vi "LED_current_stability.vi"() -> ()   [LabVIEW 2012]
uses:
  <instrlib>/Keithley 2600 Series/Public/Channel.ctl
  <vilib>/Utility/file.llb/Read From Spreadsheet File (DBL).vi
  <vilib>/Utility/file.llb/Write To Spreadsheet File (string).vi
  <vilib>/Utility/file.llb/Write To Spreadsheet File (DBL).vi
  <instrlib>/Keithley 2600 Series/Keithley 2600 Series.lvlib
  <vilib>/Analysis/NI_AALPro.lvlib
  <vilib>/gmath/NI_Gmath.lvlib
panel:
  out "CurDen array":string[](array[string])
  out "power array":string[](array[string])
  out "Power(W)":dbl
  out "DeltaWL":dbl[](array[numeric])
  out "data path":path
  out "DarkSpectrum path":path
  out "Info path":path
  out "AllSpectrum path":path
  out "EQE array":string[](array[string])
  out "LPE array":string[](array[string])
  out "CE array":string[](array[string])
  out "L/L0 array":string[](array[string])
  out "Lum array":string[](array[string])
  out "voltage array":string[](array[string])
  out "current array":string[](array[string])
  out "time array":string[](array[string])
  out "Info3":string
  out "Info2":string
  out "Info1":string
  out "time string":string
  out "date string":string
  out "Status":string
  in  "Tab Control":T1(tab)
  in  "VISA resource name":refnum<visa-resource-name>
  in  "Source Current (A)":dbl=1.1e-05 format="%#_5e"
  in  "Voltage Limit (V)":dbl=10.0
  in  "Integration Time (ms)":dbl=10.0
  in  "Interval (s)":u32=5
  in  "Initial wait (ms)":u32=2000
  in  "Calibration File":path
  in  "Dev_Area (m2)":dbl=3e-06
  in  "WL_high":dbl=785.0
  in  "WL_low":dbl=365.0
  in  "Ratio for auto stop":dbl
  in  "File Path":path
  in  "Auto stop":bool
  in  "Boxcar Width":i32
  in  "Sample description:":string="Please write here..."
  out "Measured Voltage (V)":string
  out "Measured Current (A)":string
  out "WL_2":dbl format="%#_5g"
  out "WL_1":dbl format="%#_5g"
  out "EQE (%)":dbl format="%_3e"
  out "Lum. Pow. Eff. (lm/W)":dbl format="%_3e"
  out "Lum.(cd/m2)":dbl format="%_3e"
  out "Cur. Eff. (cd/A)":dbl format="%_3e"
  out "Lum0":dbl format="%_3e"
  out "Lum/Lum0":dbl format="%_3e"
  out "Time (s)":dbl
  out "Spectra":T2(graph)
  out "Graph":cluster{dbl[], dbl[]}(graph)
  out "Measured_Current(A)":dbl format="%_3e"
  out "Measured_voltage(V)":dbl format="%_3e"
  in  "Ring":i32(ring)=1 items=["L/L0", "Lum", "C.E.", "L.P.E.", "EQE", "Power"]
  out "Maximum Intensity":i32 format="%.2e"
  out "BoxcarWidth":i32
  out "Detector Saturated":bool
  out "All Info":string
  out "VISA resource name out":refnum<visa-resource-name>
  out "error out":errorcluster
  out "x2":i32
  out "x1":i32
  out "Photon_count":dbl
  out "Energy_WL":dbl[](array[numeric])
  out "Candela":dbl
  out "Abs_Irr (W/nm)":dbl[](array[numeric])
  out "Dark_spectrum":dbl[](array[numeric])
  out "Keithley":bool
  out "Spectrometer":bool
  out "Current density (mA/cm2)":dbl
  out "Iso. Coef. itpl":dbl[](array[numeric]) format="%_6g"
  out "WL itpl":dbl[](array[numeric]) format="%_6g"
  out "EyeRespCoef.":dbl[](array[numeric])
  out "WL_EyeResp":dbl[](array[numeric])
  out "WL_cal":dbl[](array[numeric])
  out "cal_CountsToAbsIrr":dbl[](array[numeric])
  in  "Start":bool
  in  "stop":bool
  out "Measured_Spectrum":dbl[](array[numeric])
  out "Wrapper Out":u64
  out "WL_spectrometer":dbl[](array[numeric])
  out "Number of Spectrometers":i32
  out "Node Out":string
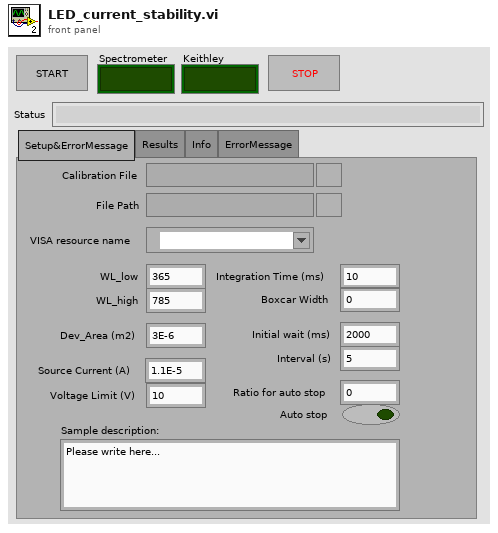
[diagram p1: front panel]
types:
  T1 = enum32{"Setup&ErrorMessage", "Results", "Info", "ErrorMessage"}
  T2 = cluster{"WL_spectrometer":dbl[], "Dark_spectrum":dbl[]}
  T3 = enum32{"Current", "Voltage", "IV", "Resistance", "Power"}
  T4 = typedef "Keithley 2600 Series.lvlib/Channel.ctl" = enum32{"Channel A", "Channel B"}
  T5 = cluster{"WL_spectrometer":dbl[], "Measured_Spectrum":dbl[]}
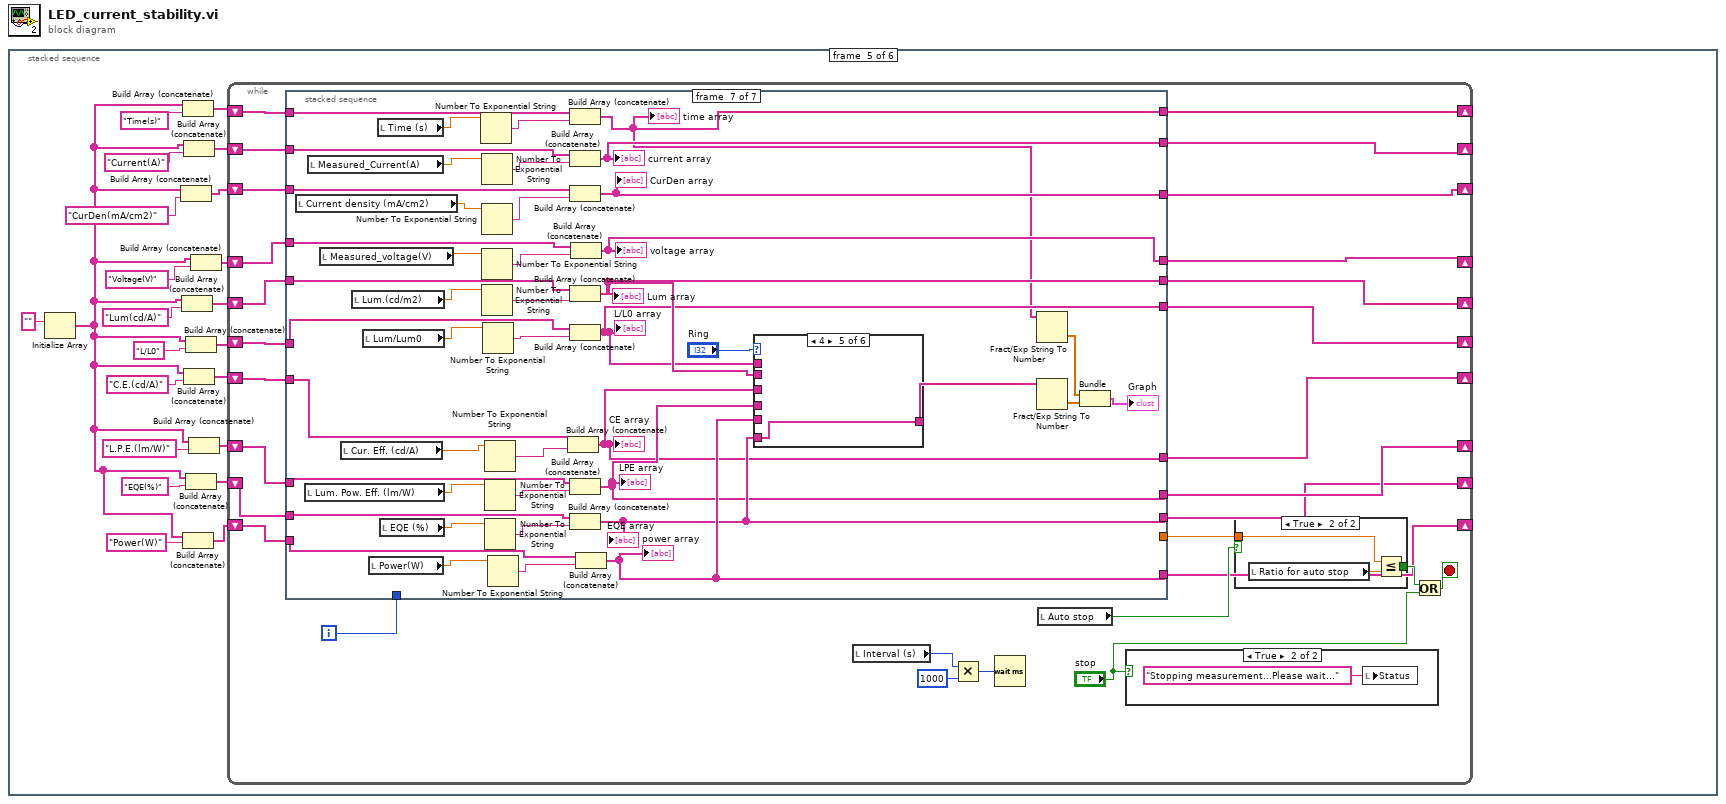
[diagram p0: block diagram]
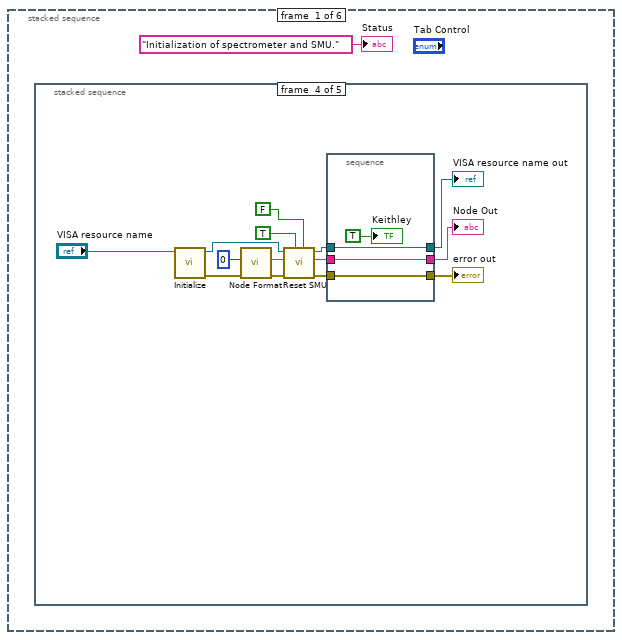
[diagram p2: hidden frame]
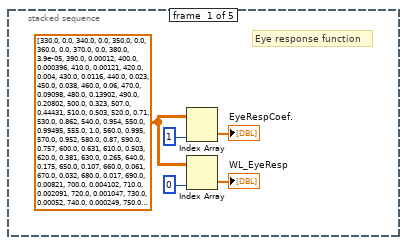
[diagram p3: hidden frame]
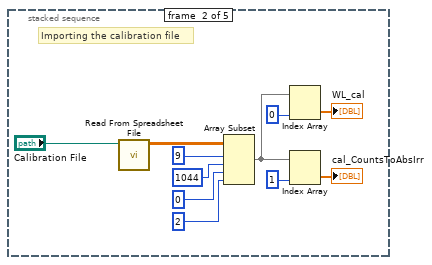
[diagram p4: hidden frame]
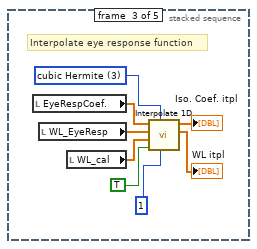
[diagram p5: hidden frame]
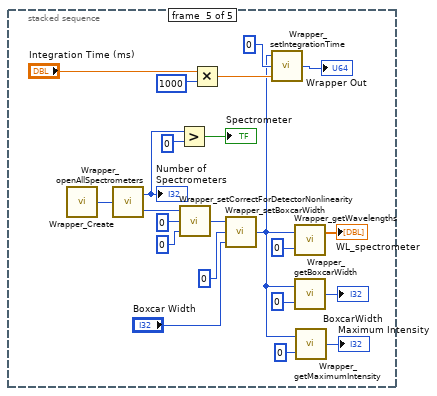
[diagram p6: hidden frame]
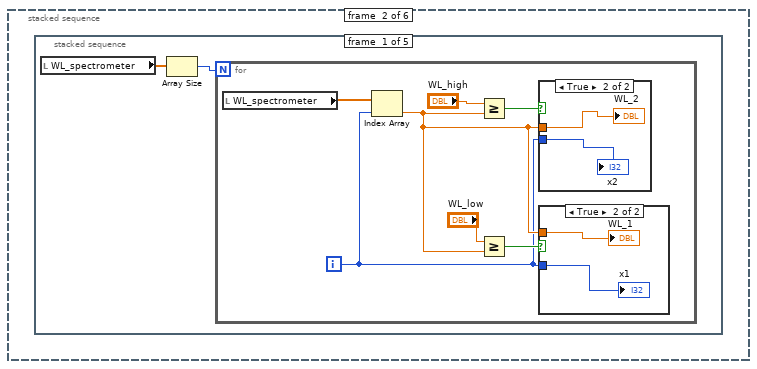
[diagram p7: hidden frame]
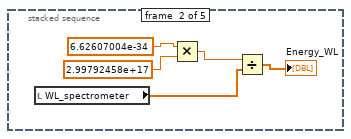
[diagram p10: hidden frame]
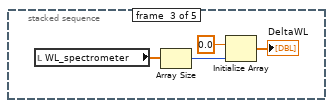
[diagram p11: hidden frame]
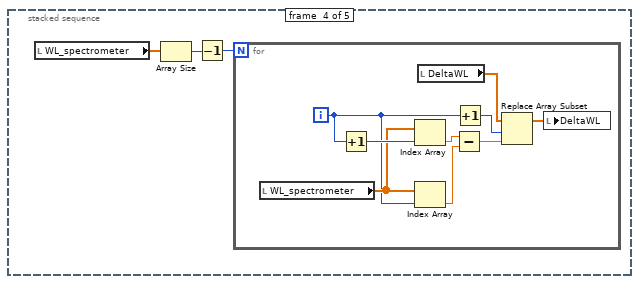
[diagram p12: hidden frame]
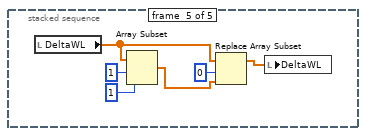
[diagram p13: hidden frame]
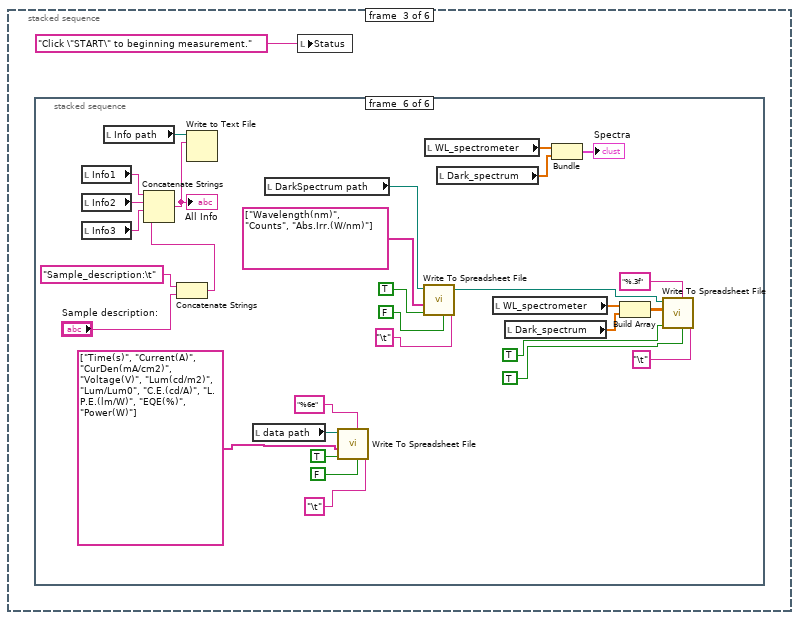
[diagram p14: hidden frame]
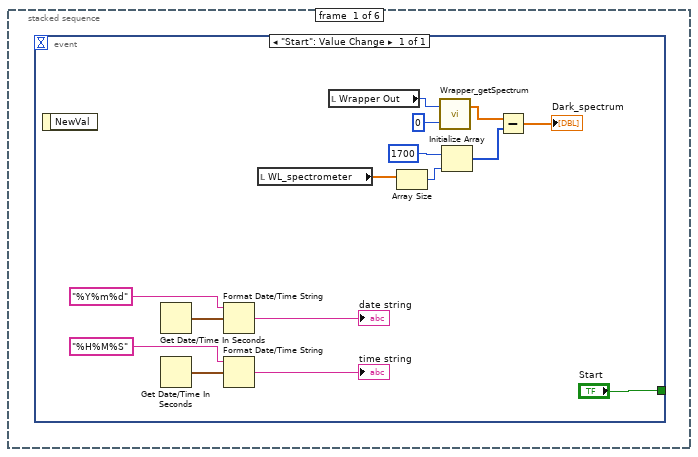
[diagram p15: hidden frame]
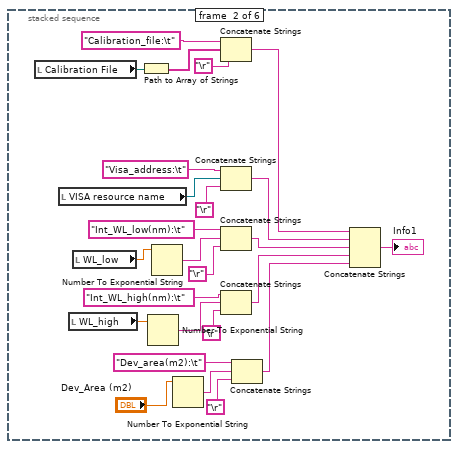
[diagram p16: hidden frame]
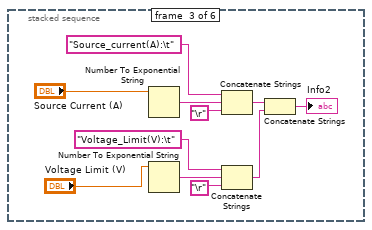
[diagram p17: hidden frame]
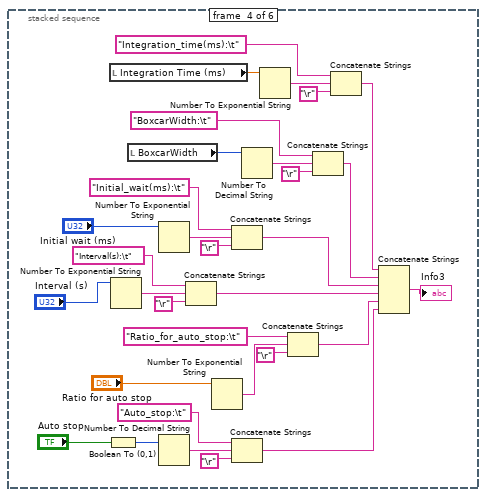
[diagram p18: hidden frame]
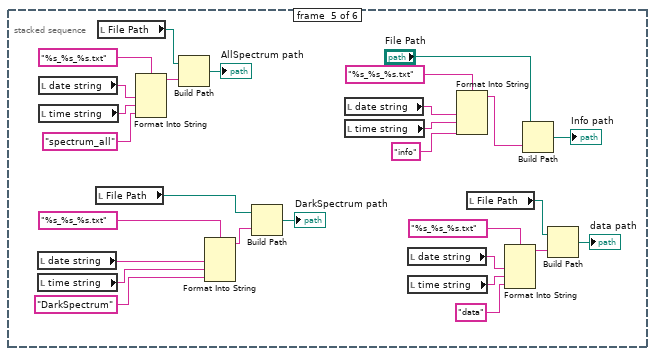
[diagram p19: hidden frame]
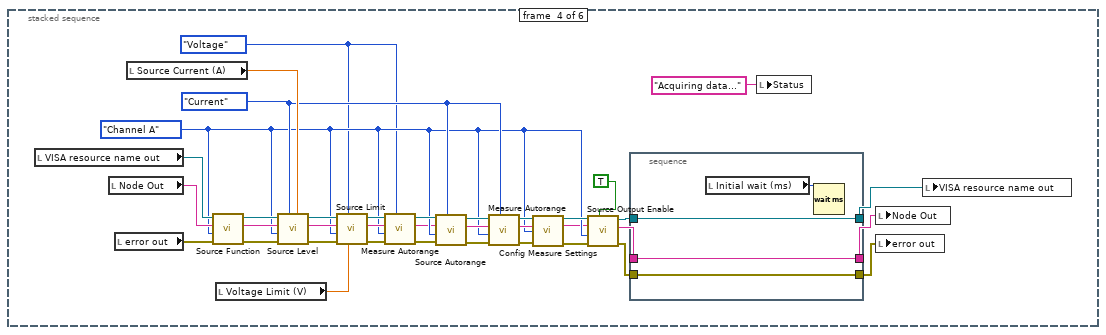
[diagram p20: hidden frame]
diagram:
  n1 = stacked-sequence {
    frame #0 {
      n2 = stacked-sequence {
        frame #0 {
          w5 = dbl[][] [[330.0, 0.0], [340.0, 0.0], [350.0, 0.0], [360.0, 0.0], [370.0, 0.0], [380.0, 3.9e-05], [390.0, 0.00012], [400.0, 0.000396], [410.0, 0.00121], [420.0, 0.004], [430.0, 0.0116], [440.0, 0.023], [450.0, 0.038], [460.0, 0.06], [470.0, 0.09098], [480.0, 0.13902], [490.0, 0.20802], [500.0, 0.323], [507.0, 0.44431], [510.0, 0.503], [520.0, 0.71], [530.0, 0.862], [540.0, 0.954], [550.0, 0.99495], [555.0, 1.0], [560.0, 0.995], [570.0, 0.952], [580.0, 0.87], [590.0, 0.757], [600.0, 0.631], [610.0, 0.503], [620.0, 0.381], [630.0, 0.265], [640.0, 0.175], [650.0, 0.107], [660.0, 0.061], [670.0, 0.032], [680.0, 0.017], [690.0, 0.00821], [700.0, 0.004102], [710.0, 0.002091], [720.0, 0.001047], [730.0, 0.00052], [740.0, 0.000249], [750.0, 0.00012], [760.0, 6e-05], [770.0, 3e-05], [780.0, 0.0], [790.0, 0.0], [800.0, 0.0], [810.0, 0.0], [820.0, 0.0], [830.0, 0.0], [840.0, 0.0], [850.0, 0.0], [860.0, 0.0], [870.0, 0.0], [880.0, 0.0], [890.0, 0.0], [900.0, 0.0], [910.0, 0.0], [920.0, 0.0], [930.0, 0.0], [940.0, 0.0], [950.0, 0.0], [960.0, 0.0], [970.0, 0.0], [980.0, 0.0], [990.0, 0.0], [1000.0, 0.0], [1010.0, 0.0], [1020.0, 0.0], [1030.0, 0.0], [1040.0, 0.0], [1050.0, 0.0], [1060.0, 0.0], [1070.0, 0.0], [1080.0, 0.0], [1090.0, 0.0], [1100.0, 0.0], [1110.0, 0.0], [1120.0, 0.0], [1130.0, 0.0], [1140.0, 0.0]] ("all rows")
          # "Eye response function"
          n3 = Index Array(array=w5, index (col)=1 ("disabled index (col)")) -> (element=→"EyeRespCoef.":dbl[])  [unwired: 1 in]
          n4 = Index Array(array=w5, index (col)=0 ("disabled index (col)")) -> (element=→"WL_EyeResp":dbl[])  [unwired: 1 in]
        }
        frame #1 {
          # "Importing the calibration file"
          n5 = call-poly <vilib>:"Read From Spreadsheet File.vi"("file path (dialog if empty)"="Calibration File") -> ("all rows"=w10:dbl[][])  [unwired: 6 in, 4 out]
          n6 = Array Subset(array=w10, index (row)=9 ("index"), length (row)=1044 ("length"), index (col)=0 ("index"), length (col)=2 ("length")) -> (w13:dbl[][])
          n7 = Index Array(array=w13, index (col)=0 ("index")) -> (element=→"WL_cal":dbl[])  [unwired: 1 in]
          n8 = Index Array(array=w13, index (col)=1 ("length")) -> (element=→"cal_CountsToAbsIrr":dbl[])  [unwired: 1 in]
        }
        frame #2 {
          w21 = 3 items=["nearest", "linear", "spline", "cubic Hermite", "Lagrange"] ("method")
          # "Interpolate eye response function"
          n9 = local read "EyeRespCoef."() -> (w24:dbl[])
          n10 = local read "WL_EyeResp"() -> (w25:dbl[])
          n11 = local read "WL_cal"() -> (w23:dbl[])
          n12 = call <vilib>:"Interpolate 1D.vi"("ntimes"=1, "method"=w21, "X is monotonic"=TRUE, "xi"=w23, "X"=w25, "Y"=w24) -> ("xi used"=→"WL itpl":dbl[], "yi"=→"Iso. Coef. itpl":dbl[])  [unwired: 3 in, 1 out]
        }
        frame #3 {
          n13 = call <instrlib>:"Initialize.vi"("VISA resource name"="VISA resource name") -> ("error out"=w37:errorcluster, "VISA resource name out"=w39:refnum<visa-resource-name>)  [unwired: 5 in, 4 out]
          n14 = call <instrlib>:"Node Format.vi"("error in"=w37, "Node (0-64)"=i8 0) -> ("error out"=w36:errorcluster, "Formatted Node"=w38:string)  [unwired: 8 out]
          n15 = call <instrlib>:"Reset SMU.vi"("SMU B (No)"=FALSE, "SMU A (No)"=TRUE, "error in (no error)"=w36, "Node In"=w38, "VISA resource name"=w39) -> ("error out"=w31:errorcluster, "Node Out"=w29:string, "VISA resource name out"=w27:refnum<visa-resource-name>)  [unwired: 4 out]
          n16 = stacked-sequence {
            tunnel: [w42] -> w30
            tunnel: w31 -> [w42]
            tunnel: w29 -> [w41]
            tunnel: [w41] -> w28
            tunnel: w27 -> [w40]
            tunnel: [w40] -> w26
            frame #0 {
              "Keithley" <- TRUE ("Keithley")
            }
          }
          "Node Out" <- w28
          "error out" <- w30
          "VISA resource name out" <- w26
        }
        frame #4 {
          n17 = call "Wrapper_Create.vi"() -> ("Wrapper"=w65:u64)
          n18 = call "Wrapper_openAllSpectrometers.vi"("Wrapper In"=w65) -> ("Number of Spectrometers"=w58:i32, "Wrapper Out"=w49:u64)
          "Number of Spectrometers" <- w58
          n19 = Greater?(x=w58, y=0) -> (0:→"Spectrometer":bool)
          n20 = call "Wrapper_setCorrectForDetectorNonlinearity.vi"("On/Off"=0, "Index"=0, "Wrapper In"=w49) -> ("Wrapper Out"=w54:u64)
          n21 = Multiply(x="Integration Time (ms)", y=1000) -> (x*y=w61:dbl)
          n22 = call "Wrapper_setBoxcarWidth.vi"("Boxcar Width"="Boxcar Width", "Index"=0, "Wrapper In"=w54) -> ("Wrapper Out"=w48:u64)
          n23 = call "Wrapper_setIntegrationTime.vi"("Integration Time"=w61, "Index"=0, "Wrapper In"=w48) -> ("Wrapper Out"=→"Wrapper Out":u64)
          n24 = call "Wrapper_getWavelengths.vi"("Index"=0, "Wrapper"=w48) -> ("WL Values"=→"WL_spectrometer":dbl[])  [unwired: 1 out]
          n25 = call "Wrapper_getBoxcarWidth.vi"("Index"=0, "Wrapper"=w48) -> ("BoxcarWidth"=→"BoxcarWidth":i32)
          n26 = call "Wrapper_getMaximumIntensity.vi"("Index"=0, "Wrapper"=w48) -> ("Maximum Intensity"=→"Maximum Intensity":i32)
        }
      }
      "Status" <- "Initialization of spectrometer and SMU." ("Measured Current (A) 2")
    }
    frame #1 {
      n27 = stacked-sequence {
        frame #0 {
          n28 = local read "WL_spectrometer"() -> (w66:dbl[])
          n29 = Array Size(array=w66) -> (size(s)=w67:i32)
          n30 = for {
            N: w67 -> [_]
            i -> [w68]
            n31 = local read "WL_spectrometer"() -> (w70:dbl[])
            n32 = Index Array(array=w70, index=w68) -> (element=w69:dbl)
            n33 = Greater Or Equal?(x="WL_high", y=w69) -> (x >= y?=w72:bool)
            n34 = Greater Or Equal?(x="WL_low", y=w69) -> (x >= y?=w71:bool)
            n35 = case shown="True" w72 {
              tunnel: w69 -> [_ w77]
              tunnel: w68 -> [_ w78]
              frame False {
              }
              frame True {
                "WL_2" <- w77
                "x2" <- w78
              }
            }
            n36 = case shown="True" w71 {
              tunnel: w69 -> [_ w75]
              tunnel: w68 -> [_ w76]
              frame False {
              }
              frame True {
                "WL_1" <- w75
                "x1" <- w76
              }
            }
          }
        }
        frame #1 {
          n37 = local read "WL_spectrometer"() -> (w82:dbl[])
          n38 = Multiply(x=6.62607004e-34, y=2.99792458e+17) -> (x*y=w81:dbl)
          n39 = Divide(x=w81, y=w82) -> (x/y=→"Energy_WL":dbl[])
        }
        frame #2 {
          n40 = local read "WL_spectrometer"() -> (w87:dbl[])
          n41 = Array Size(array=w87) -> (size(s)=w85:i32)
          n42 = Initialize Array(0.0, w85) -> (→"DeltaWL":dbl[])
        }
        frame #3 {
          n43 = local read "WL_spectrometer"() -> (w90:dbl[])
          n44 = Array Size(array=w90) -> (size(s)=w89:i32)
          n45 = Decrement(x=w89) -> (x-1=w88:i32)
          n46 = for {
            N: w88 -> [_]
            i -> [w95]
            n47 = local read "WL_spectrometer"() -> (w98:dbl[])
            n48 = Increment(x=w95) -> (x+1=w99:i32)
            n49 = Index Array(array=w98, index=w99) -> (element=w97:dbl)
            n50 = Index Array(array=w98, index=w95) -> (element=w96:dbl)
            n51 = local read "DeltaWL"() -> (w92:dbl[])
            n52 = Subtract(x=w97, y=w96) -> (x-y=w93:dbl)
            n53 = Increment(x=w95) -> (x+1=w94:i32)
            n54 = Replace Array Subset(array=w92, new element=w93, index=w94) -> (w91:dbl[])
            n55 = local write "DeltaWL"(w91) -> ()
          }
        }
        frame #4 {
          n56 = local read "DeltaWL"() -> (w100:dbl[])
          n57 = Array Subset(array=w100, index=1, length=1) -> (w101:dbl[])
          n58 = Replace Array Subset(array=w100, new element=w101, index=0) -> (w105:dbl[])
          n59 = local write "DeltaWL"(w105) -> ()
        }
      }
    }
    frame #2 {
      n60 = stacked-sequence {
        frame #0 {
          n61 = event shown="[0] \"Start\": Value Change" {
            selector: _ -> [_]
            dyn-events: _ -> [_]
            timeout: _ -> [_]
            tunnel: ["Start"] -> _
            event "Start": Value Change {
              n62 = event-data() -> ()  [unwired: 1 in, 1 out]
              n63 = Get Date/Time In Seconds() -> (seconds since 1Jan1904=w119:timestamp)
              n64 = Get Date/Time In Seconds() -> (seconds since 1Jan1904=w117:timestamp)
              n65 = Format Date/Time String(time format string (%c)="%Y%m%d" ("Timestamp string format i%cj"), seconds (now)=w119) -> (date/time string=→"date string":string)  [unwired: 1 out]
              n66 = Format Date/Time String(time format string (%c)="%H%M%S" ("Timestamp string format i%cj"), seconds (now)=w117) -> (date/time string=→"time string":string)  [unwired: 1 out]
              n67 = local read "WL_spectrometer"() -> (w112:dbl[])
              n68 = local read "Wrapper Out"() -> (w113:u64)
              n69 = Array Size(array=w112) -> (size(s)=w111:i32)
              n70 = call "Wrapper_getSpectrum.vi"("Index"=0, "Wrapper"=w113) -> ("Spectrum Values"=w109:dbl[])  [unwired: 1 out]
              n71 = Initialize Array(1700, w111) -> (w108:i32[])
              n72 = Subtract(x=w109, y=w108) -> (x-y=→"Dark_spectrum":dbl[])
            }
          }
        }
        frame #1 {
          n73 = local read "Calibration File"() -> (w123:path)
          n74 = local read "VISA resource name"() -> (w129:refnum<visa-resource-name>)
          n75 = local read "WL_high"() -> (w125:dbl)
          n76 = local read "WL_low"() -> (w124:dbl)
          n77 = Path to Array of Strings(0:w123) -> (2:w127:string[])  [unwired: 1 out]
          n78 = Number To Exponential String(number=w125) -> (E-format string=w133:string)  [unwired: 3 in]
          n79 = Number To Exponential String(number=w124) -> (E-format string=w130:string)  [unwired: 3 in]
          n80 = Number To Exponential String(number="Dev_Area (m2)") -> (E-format string=w136:string)  [unwired: 3 in]
          n81 = Concatenate Strings("Calibration_file:\t" ("string"), w127, "\r") -> (w137:string)
          n82 = Concatenate Strings("Visa_address:\t" ("string"), w129, "\r") -> (w138:string)
          n83 = Concatenate Strings("Int_WL_low(nm):\t" ("string"), w130, "\r") -> (w139:string)
          n84 = Concatenate Strings("Int_WL_high(nm):\t" ("string"), w133, "\r") -> (w140:string)
          n85 = Concatenate Strings("Dev_area(m2):\t" ("string"), w136, "\r") -> (w141:string)
          n86 = Concatenate Strings(w137, w138, w139, w140, w141) -> (→"Info1":string)
        }
        frame #2 {
          n87 = Number To Exponential String(number="Source Current (A)") -> (E-format string=w149:string)  [unwired: 3 in]
          n88 = Number To Exponential String(number="Voltage Limit (V)") -> (E-format string=w152:string)  [unwired: 3 in]
          n89 = Concatenate Strings("Source_current(A):\t" ("string"), w149, "\r") -> (w154:string)
          n90 = Concatenate Strings("Voltage_Limit(V):\t" ("string"), w152, "\r") -> (w155:string)
          n91 = Concatenate Strings(w154, w155) -> (→"Info2":string)
        }
        frame #3 {
          n92 = Boolean To (0,1)(Boolean="Auto stop") -> (0, 1=w166:i16)
          n93 = local read "Integration Time (ms)"() -> (w177:dbl)
          n94 = Number To Exponential String(number="Interval (s)") -> (E-format string=w183:string)  [unwired: 3 in]
          n95 = local read "BoxcarWidth"() -> (w159:i32)
          n96 = Number To Exponential String(number="Initial wait (ms)") -> (E-format string=w179:string)  [unwired: 3 in]
          n97 = Number To Decimal String(number=w166) -> (decimal integer string=w165:string)  [unwired: 1 in]
          n98 = Concatenate Strings("Interval(s):\t" ("string"), w183, "\r") -> (w188:string)
          n99 = Number To Exponential String(number="Ratio for auto stop") -> (E-format string=w184:string)  [unwired: 3 in]
          n100 = Concatenate Strings("Initial_wait(ms):\t" ("string"), w179, "\r") -> (w187:string)
          n101 = Concatenate Strings("Auto_stop:\t" ("string"), w165, "\r") -> (w164:string)
          n102 = Number To Decimal String(number=w159) -> (decimal integer string=w163:string)  [unwired: 1 in]
          n103 = Number To Exponential String(number=w177) -> (E-format string=w176:string)  [unwired: 3 in]
          n104 = Concatenate Strings("Ratio_for_auto_stop:\t" ("string"), w184, "\r") -> (w189:string)
          n105 = Concatenate Strings("BoxcarWidth:\t" ("string"), w163, "\r") -> (w161:string)
          n106 = Concatenate Strings("Integration_time(ms):\t" ("string"), w176, "\r") -> (w160:string)
          n107 = Concatenate Strings(w160, w161, w187, w188, w189, w164) -> (→"Info3":string)
        }
        frame #4 {
          n108 = local read "date string"() -> (w203:string)
          n109 = local read "time string"() -> (w204:string)
          n110 = local read "date string"() -> (w214:string)
          n111 = local read "time string"() -> (w215:string)
          n112 = local read "File Path"() -> (w202:path)
          n113 = local read "File Path"() -> (w216:path)
          n114 = Format Into String(format string="%s_%s_%s.txt" ("Format string"), w214, w215, "spectrum_all" ("input 2")) -> (resulting string=w213:string)  [unwired: 2 in, 1 out]
          n115 = Build Path(base path=w216, name or relative path=w213) -> (appended path=→"AllSpectrum path":path)
          n116 = Format Into String(format string="%s_%s_%s.txt" ("Format string"), w203, w204, "DarkSpectrum" ("input 2")) -> (resulting string=w201:string)  [unwired: 2 in, 1 out]
          n117 = Build Path(base path=w202, name or relative path=w201) -> (appended path=→"DarkSpectrum path":path)
          n118 = local read "date string"() -> (w207:string)
          n119 = local read "time string"() -> (w209:string)
          n120 = local read "date string"() -> (w192:string)
          n121 = local read "time string"() -> (w193:string)
          n122 = Format Into String(format string="%s_%s_%s.txt" ("Format string"), w207, w209, "info" ("input 2")) -> (resulting string=w210:string)  [unwired: 2 in, 1 out]
          n123 = local read "File Path"() -> (w195:path)
          n124 = Format Into String(format string="%s_%s_%s.txt" ("Format string"), w192, w193, "data" ("input 2")) -> (resulting string=w191:string)  [unwired: 2 in, 1 out]
          n125 = Build Path(base path="File Path", name or relative path=w210) -> (appended path=→"Info path":path)
          n126 = Build Path(base path=w195, name or relative path=w191) -> (appended path=→"data path":path)
        }
        frame #5 {
          n127 = local read "Info1"() -> (w246:string)
          n128 = local read "Info2"() -> (w245:string)
          n129 = local read "Info3"() -> (w244:string)
          n130 = local read "Info path"() -> (w233:path)
          n131 = Concatenate Strings("Sample_description:\t" ("string"), "Sample description:") -> (w218:string)
          n132 = Concatenate Strings(w246, w245, w244, w218) -> (w247:string)
          "All Info" <- w247
          n133 = Write to Text File(file (use dialog)=w233, text=w247) -> ()  [unwired: 2 in, 3 out]
          n134 = local read "data path"() -> (w226:path)
          n135 = local read "DarkSpectrum path"() -> (w228:path)
          n136 = call-poly <vilib>:"Write To Spreadsheet File.vi"("delimiter (\\t)"="\t" ("delimiter (\\t)"), "transpose? (no:F)"=FALSE, "format (%s)"="%6e" ("format (%.3f)"), "append to file? (new file:F)"=TRUE, "1D data"=string[] ["Time(s)", "Current(A)", "CurDen(mA/cm2)", "Voltage(V)", "Lum(cd/m2)", "Lum/Lum0", "C.E.(cd/A)", "L.P.E.(lm/W)", "EQE(%)", "Power(W)"], "file path (dialog if empty)"=w226) -> ()  [unwired: 1 in, 2 out]
          n137 = call-poly <vilib>:"Write To Spreadsheet File.vi"("delimiter (\\t)"="\t" ("delimiter (\\t)"), "transpose? (no:F)"=FALSE, "append to file? (new file:F)"=TRUE, "1D data"=string[] ["Wavelength(nm)", "Counts", "Abs.Irr.(W/nm)"], "file path (dialog if empty)"=w228) -> ("new file path (Not A Path if cancelled)"=w227:path)  [unwired: 2 in, 1 out]
          n138 = local read "WL_spectrometer"() -> (w234:dbl[])
          n139 = local read "Dark_spectrum"() -> (w235:dbl[])
          n140 = local read "WL_spectrometer"() -> (w238:dbl[])
          n141 = local read "Dark_spectrum"() -> (w237:dbl[])
          n142 = Bundle("WL_spectrometer"=w234, "Dark_spectrum"=w235) -> (→"Spectra":T2)  [unwired: 1 in]
          n143 = Build Array(w238, w237) -> (w239:dbl[][])
          n144 = call-poly <vilib>:"Write To Spreadsheet File.vi"("delimiter (\\t)"="\t" ("delimiter (\\t)"), "transpose? (no:F)"=TRUE, "format (%.3f)"="%.3f", "append to file? (new file:F)"=TRUE, "2D data"=w239, "file path (dialog if empty)"=w227) -> ()  [unwired: 1 in, 2 out]
        }
      }
      n145 = local write "Status"("Click \"START\" to beginning measurement." ("Status")) -> ()
    }
    frame #3 {
      w251 = enum32{"Current", "Voltage"}."Voltage" ("Function (Current)")
      w257 = enum32{"Current", "Voltage"}."Current" ("Function (Current)")
      w252 = Channel."Channel A" ("Channel (Channel A)")
      n146 = local read "VISA resource name out"() -> (w276:refnum<visa-resource-name>)
      n147 = local read "Node Out"() -> (w277:string)
      n148 = local read "error out"() -> (w278:errorcluster)
      n149 = local read "Source Current (A)"() -> (w268:dbl)
      n150 = call <instrlib>:"Source Function.vi"("error in (no error)"=w278, "Channel (Channel A)"=w252, "Node In"=w277, "VISA resource name"=w276) -> ("error out"=w281:errorcluster, "Node Out"=w279:string, "VISA resource name out"=w280:refnum<visa-resource-name>)  [unwired: 1 in, 4 out]
      n151 = local read "Voltage Limit (V)"() -> (w267:dbl)
      n152 = call <instrlib>:"Source Level.vi"("Level (0.000)"=w268, "Function (Current)"=w257, "error in (no error)"=w281, "Channel (Channel A)"=w252, "Node In"=w279, "VISA resource name"=w280) -> ("error out"=w282:errorcluster, "Node Out"=w284:string, "VISA resource name out"=w283:refnum<visa-resource-name>)  [unwired: 3 out]
      n153 = call <instrlib>:"Source Limit.vi"("Limit (0.000)"=w267, "Function (Current)"=w251, "error in (no error)"=w282, "Channel (Channel A)"=w252, "Node In"=w284, "VISA resource name"=w283) -> ("error out"=w260:errorcluster, "Node Out"=w259:string, "VISA resource name out"=w258:refnum<visa-resource-name>)  [unwired: 3 out]
      n154 = call <instrlib>:"Measure Autorange.vi"("Function (Current)"=w251, "error in (no error)"=w260, "Channel (Channel A)"=w252, "Node In"=w259, "VISA resource name"=w258) -> ("error out"=w256:errorcluster, "Node Out"=w250:string, "VISA resource name out"=w255:refnum<visa-resource-name>)  [unwired: 1 in, 3 out]
      n155 = call <instrlib>:"Source Autorange.vi"("Function (Current)"=w257, "error in (no error)"=w256, "Channel (Channel A)"=w252, "Node In"=w250, "VISA resource name"=w255) -> ("error out"=w264:errorcluster, "Node Out"=w261:string, "VISA resource name out"=w265:refnum<visa-resource-name>)  [unwired: 1 in, 3 out]
      n156 = call <instrlib>:"Measure Autorange.vi"("Function (Current)"=w257, "error in (no error)"=w264, "Channel (Channel A)"=w252, "Node In"=w261, "VISA resource name"=w265) -> ("error out"=w263:errorcluster, "Node Out"=w262:string, "VISA resource name out"=w266:refnum<visa-resource-name>)  [unwired: 1 in, 3 out]
      n157 = call <instrlib>:"Config Measure Settings.vi"("VISA resource name"=w266, "Node In"=w262, "Channel (Channel A)"=w252, "error in"=w263) -> ("VISA resource name out"=w253:refnum<visa-resource-name>, "Node Out"=w249:string, "error out"=w254:errorcluster)  [unwired: 6 in, 3 out]
      n158 = call <instrlib>:"Source Output Enable.vi"("Output (Off)"=TRUE, "error in (no error)"=w254, "Channel (Channel A)"=w252, "Node In"=w249, "VISA resource name"=w253) -> ("error out"=w274:errorcluster, "Node Out"=w273:string, "VISA resource name out"=w272:refnum<visa-resource-name>)  [unwired: 4 out]
      n159 = stacked-sequence {
        tunnel: w274 -> [w288]
        tunnel: [w288] -> w269
        tunnel: w273 -> [w287]
        tunnel: [w287] -> w270
        tunnel: w272 -> [w286]
        tunnel: [w286] -> w271
        frame #0 {
          n160 = local read "Initial wait (ms)"() -> (w285:u32)
          n161 = Wait (ms)(milliseconds to wait=w285) -> ()  [unwired: 1 out]
        }
      }
      n162 = local write "Status"("Acquiring data..." ("Status")) -> ()
      n163 = local write "Node Out"(w270) -> ()
      n164 = local write "error out"(w269) -> ()
      n165 = local write "VISA resource name out"(w271) -> ()
    }
    frame #4 {
      n166 = Initialize Array("" ("element")) -> (w291:string[])  [unwired: 1 in]
      n167 = Build Array (concatenate)(w291, "CurDen(mA/cm2)" ("Status")) -> (w289:string[])
      n168 = Build Array (concatenate)(w291, "Lum(cd/A)" ("Status")) -> (w298:string[])
      n169 = Build Array (concatenate)(w291, "Time(s)" ("Status")) -> (w295:string[])
      n170 = Build Array (concatenate)(w291, "Power(W)" ("Status")) -> (w290:string[])
      n171 = Build Array (concatenate)(w291, "Current(A)" ("Status")) -> (w296:string[])
      n172 = Build Array (concatenate)(w291, "C.E.(cd/A)" ("Status")) -> (w300:string[])
      n173 = Build Array (concatenate)(w291, "L/L0" ("Status")) -> (w299:string[])
      n174 = Build Array (concatenate)(w291, "EQE(%)" ("Status")) -> (w302:string[])
      n175 = Build Array (concatenate)(w291, "L.P.E.(lm/W)" ("Status")) -> (w301:string[])
      n176 = Build Array (concatenate)(w291, "Voltage(V)" ("Status")) -> (w297:string[])
      n177 = while {
        shift-right: [w325] -> _
        shift-left: w295 -> [w333]
        shift-right: [w324] -> _
        shift-left: w296 -> [w332]
        shift-right: [w323] -> _
        shift-left: w297 -> [w331]
        shift-right: [w322] -> _
        shift-left: w298 -> [w330]
        shift-right: [w321] -> _
        shift-left: w299 -> [w329]
        shift-right: [w320] -> _
        shift-left: w300 -> [w328]
        shift-right: [w318] -> _
        shift-left: w302 -> [w326]
        shift-right: [w319] -> _
        shift-left: w301 -> [w327]
        shift-right: [w315] -> _
        shift-left: w290 -> [w316]
        shift-right: [w313] -> _
        shift-left: w289 -> [w314]
        i -> [w337]
        stop <- w336 stop-if-true
        n178 = stacked-sequence {
          tunnel: w337 -> [_ _ _ w448 _ _ _]
          tunnel: w333 -> [_ _ _ _ _ _ w530]
          tunnel: w332 -> [_ _ _ _ _ _ w529]
          tunnel: w331 -> [_ _ _ _ _ _ w528]
          tunnel: w330 -> [_ _ _ _ _ _ w527]
          tunnel: w329 -> [_ _ _ _ _ _ w526]
          tunnel: w328 -> [_ _ _ _ _ _ w525]
          tunnel: w327 -> [_ _ _ _ _ _ w524]
          tunnel: w326 -> [_ _ _ _ _ _ w523]
          tunnel: [_ _ _ _ _ _ w486] -> w325
          tunnel: [_ _ _ _ _ _ w500] -> w324
          tunnel: [_ _ _ _ _ _ w498] -> w323
          tunnel: [_ _ _ _ _ _ w488] -> w322
          tunnel: [_ _ _ _ _ _ w487] -> w321
          tunnel: [_ _ _ _ _ _ w489] -> w320
          tunnel: [_ _ _ _ _ _ w490] -> w319
          tunnel: [_ _ _ _ _ _ w491] -> w318
          tunnel: w316 -> [_ _ _ _ _ _ w504]
          tunnel: [_ _ _ _ _ _ w492] -> w315
          tunnel: w314 -> [_ _ _ _ _ _ w501]
          tunnel: [_ _ _ _ _ _ w499] -> w313
          tunnel: [_ _ _ _ w467 _ _] -> w312
          frame #0 {
            w363 = Channel."Channel A" ("Channel (Channel A)")
            n179 = local read "VISA resource name out"() -> (w360:refnum<visa-resource-name>)
            n180 = local read "Node Out"() -> (w361:string)
            n181 = local read "error out"() -> (w362:errorcluster)
            n182 = local read "Wrapper Out"() -> (w351:u64)
            n183 = local read "WL_spectrometer"() -> (w348:dbl[])
            n184 = call "Wrapper_getSpectrum.vi"("Index"=0, "Wrapper"=w351) -> ("Spectrum Values"=w346:dbl[])  [unwired: 1 out]
            n185 = Array Size(array=w348) -> (size(s)=w349:i32)
            n186 = call <instrlib>:"Measure.vi"("Function (Current)"=T3."Voltage", "error in (no error)"=w362, "Channel (Channel A)"=w363, "Node In"=w361, "VISA resource name"=w360) -> ("error out"=w371:errorcluster, "Output"=w353:string, "Node Out"=w370:string, "VISA resource name out"=w369:refnum<visa-resource-name>)  [unwired: 2 in, 1 out]
            "Measured Voltage (V)" <- w353
            n187 = Initialize Array(1700, w349) -> (w347:i32[])
            n188 = Fract/Exp String To Number(string=w353) -> (number=→"Measured_voltage(V)":dbl)  [unwired: 3 in, 1 out]
            n189 = Subtract(x=w346, y=w347) -> (x-y=→"Measured_Spectrum":dbl[])
            n190 = call <instrlib>:"Measure.vi"("Function (Current)"=T3."Current", "error in (no error)"=w371, "Channel (Channel A)"=w363, "Node In"=w370, "VISA resource name"=w369) -> ("error out"=w365:errorcluster, "Output"=w356:string, "Node Out"=w367:string, "VISA resource name out"=w366:refnum<visa-resource-name>)  [unwired: 2 in, 1 out]
            "Measured Current (A)" <- w356
            n191 = local write "VISA resource name out"(w366) -> ()
            n192 = local write "Node Out"(w367) -> ()
            n193 = local write "error out"(w365) -> ()
            n194 = local read "Dev_Area (m2)"() -> (w352:dbl)
            n195 = Fract/Exp String To Number(string=w356) -> (number=w357:dbl)  [unwired: 3 in, 1 out]
            "Measured_Current(A)" <- w357
            n196 = Divide(x=w357, y=w352) -> (x/y=w358:dbl)
            n197 = Multiply(x=w358, y=0.1) -> (x*y=→"Current density (mA/cm2)":dbl)
          }
          frame #1 {
            n198 = local read "Integration Time (ms)"() -> (w412:dbl)
            n199 = local read "Measured_Spectrum"() -> (w406:dbl[])
            n200 = local read "Measured_Spectrum"() -> (w415:dbl[])
            n201 = local read "WL_spectrometer"() -> (w375:dbl[])
            n202 = local read "cal_CountsToAbsIrr"() -> (w408:dbl[])
            n203 = local read "WL_spectrometer"() -> (w405:dbl[])
            n204 = local read "Dark_spectrum"() -> (w414:dbl[])
            n205 = Bundle("WL_spectrometer"=w405, "Measured_Spectrum"=w406) -> (w407:T5)  [unwired: 1 in]
            n206 = Subtract(x=w415, y=w414) -> (x-y=w409:dbl[])
            n207 = local write "Spectra"(w407) -> ()
            n208 = local read "x2"() -> (w388:i32)
            n209 = local read "x1"() -> (w387:i32)
            n210 = local read "WL_spectrometer"() -> (w385:dbl[])
            n211 = local read "x2"() -> (w386:i32)
            n212 = local read "x1"() -> (w383:i32)
            n213 = Multiply(x=w412, y=0.001) -> (x*y=w413:dbl)
            n214 = local read "DeltaWL"() -> (w403:dbl[])
            n215 = Divide(x=w409, y=w413) -> (x/y=w410:dbl[])
            n216 = local read "Energy_WL"() -> (w397:dbl[])
            n217 = Multiply(x=w408, y=w410) -> (x*y=w404:dbl[])
            n218 = Subtract(x=w388, y=w387) -> (x-y=w393:i32)
            n219 = Subtract(x=w386, y=w383) -> (x-y=w390:i32)
            n220 = Divide(x=w404, y=w403) -> (x/y=w402:dbl[])
            n221 = Increment(x=w393) -> (x+1=w392:i32)
            n222 = Divide(x=w402, y=1000000.0) -> (x/y=w373:dbl[])
            "Abs_Irr (W/nm)" <- w373
            n223 = Increment(x=w390) -> (x+1=w389:i32)
            n224 = Divide(x=w373, y=w397) -> (x/y=w394:dbl[])
            n225 = local read "Wrapper Out"() -> (w400:u64)
            n226 = local read "Measured_Current(A)"() -> (w377:dbl)
            n227 = call <vilib>:"Uneven Numeric Integration.vi"("T"=w375, "X"=w373) -> ("result"=→"Power(W)":dbl)  [unwired: 8 in, 1 out]
            n228 = Array Subset(array=w394, index=w387, length=w392) -> (w391:dbl[])
            n229 = Array Subset(array=w385, index=w383, length=w389) -> (w384:dbl[])
            n230 = call <vilib>:"Uneven Numeric Integration.vi"("T"=w384, "X"=w391) -> ("result"=w396:dbl)  [unwired: 8 in, 1 out]
            n231 = call "Wrapper_isSaturated.vi"("Index"=0, "Wrapper"=w400) -> ("Is Saturated?"=w398:u8)
            n232 = Multiply(x=w396, y=100.0) -> (x*y=w378:dbl)
            "Photon_count" <- w378
            n233 = Divide(x=w377, y=1.60217662e-19) -> (x/y=w379:dbl)
            n234 = case shown="0, Default" w398 {
              frame 0, Default {
                "Detector Saturated" <- FALSE
              }
              frame 1 {
                n235 = local write "Detector Saturated"(TRUE ("Det.Sat.")) -> ()
              }
            }
            n236 = Divide(x=w378, y=w379) -> (x/y=w382:dbl)
            n237 = Divide(x=w382, y=3.152) -> (x/y=→"EQE (%)":dbl)
          }
          frame #2 {
            n238 = local read "Measured_Spectrum"() -> (w441:dbl[])
            n239 = local read "Iso. Coef. itpl"() -> (w421:dbl[])
            n240 = local read "Abs_Irr (W/nm)"() -> (w420:dbl[])
            n241 = local read "WL_spectrometer"() -> (w419:dbl[])
            n242 = local read "AllSpectrum path"() -> (w436:path)
            n243 = local read "WL_spectrometer"() -> (w442:dbl[])
            n244 = local read "Abs_Irr (W/nm)"() -> (w440:dbl[])
            n245 = Multiply(x=w421, y=w420) -> (x*y=w422:dbl[])
            n246 = call <vilib>:"Uneven Numeric Integration.vi"("T"=w419, "X"=w422) -> ("result"=w423:dbl)  [unwired: 8 in, 1 out]
            n247 = call-poly <vilib>:"Write To Spreadsheet File.vi"("delimiter (\\t)"="\t" ("delimiter (\\t)"), "transpose? (no:F)"=FALSE, "append to file? (new file:F)"=TRUE, "1D data"=string[] ["Wavelength(nm)", "Counts", "Abs.Irr.(W/nm)"], "file path (dialog if empty)"=w436) -> ("new file path (Not A Path if cancelled)"=w434:path)  [unwired: 2 in, 1 out]
            n248 = Build Array(w442, w441, w440) -> (w443:dbl[][])
            n249 = call-poly <vilib>:"Write To Spreadsheet File.vi"("delimiter (\\t)"="\t" ("delimiter (\\t)"), "transpose? (no:F)"=TRUE, "format (%.3f)"="%6e", "append to file? (new file:F)"=TRUE, "2D data"=w443, "file path (dialog if empty)"=w434) -> ("new file path (Not A Path if cancelled)"=w430:path)  [unwired: 1 in, 1 out]
            n250 = Multiply(x=w423, y=683.002) -> (x*y=w428:dbl)
            n251 = Multiply(x=3.141592653589793, y=3.152) -> (x*y=w424:dbl)
            n252 = Divide(x=w428, y=w424) -> (x/y=→"Candela":dbl)
            n253 = call-poly <vilib>:"Write To Spreadsheet File.vi"("delimiter (\\t)"="\t" ("delimiter (\\t)"), "transpose? (no:F)"=TRUE, "append to file? (new file:F)"=TRUE, "1D data"=string[] ["", "", "", " "], "file path (dialog if empty)"=w430) -> ()  [unwired: 2 in, 2 out]
          }
          frame #3 {
            n254 = local read "Interval (s)"() -> (w449:u32)
            n255 = local read "Dev_Area (m2)"() -> (w460:dbl)
            n256 = local read "Measured_Current(A)"() -> (w458:dbl)
            n257 = local read "Measured_Current(A)"() -> (w455:dbl)
            n258 = local read "Measured_voltage(V)"() -> (w454:dbl)
            n259 = local read "Candela"() -> (w461:dbl)
            n260 = Multiply(x=w449, y=w448) -> (x*y=→"Time (s)":u32)
            n261 = local read "Candela"() -> (w459:dbl)
            n262 = local read "Candela"() -> (w457:dbl)
            n263 = Divide(x=w461, y=w460) -> (x/y=w451:dbl)
            "Lum.(cd/m2)" <- w451
            n264 = Divide(x=w459, y=w458) -> (x/y=→"Cur. Eff. (cd/A)":dbl)
            n265 = Multiply(x=w454, y=w455) -> (x*y=w463:dbl)
            n266 = Multiply(x=w457, y=3.141592653589793) -> (x*y=w464:dbl)
            n267 = Equal?(x=0, y=w448) -> (x = y?=w452:bool)
            n268 = Divide(x=w464, y=w463) -> (x/y=→"Lum. Pow. Eff. (lm/W)":dbl)
            n269 = case shown="True" w452 {
              tunnel: w451 -> [_ w466]
              frame False {
              }
              frame True {
                "Lum0" <- w466
              }
            }
          }
          frame #4 {
            n270 = local read "Lum.(cd/m2)"() -> (w468:dbl)
            n271 = local read "Lum0"() -> (w469:dbl)
            n272 = Divide(x=w468, y=w469) -> (x/y=w467:dbl)
            "Lum/Lum0" <- w467
          }
          frame #5 {
            n273 = local read "Current density (mA/cm2)"() -> (w471:dbl)
            n274 = local read "Measured_Current(A)"() -> (w472:dbl)
            n275 = local read "Lum. Pow. Eff. (lm/W)"() -> (w477:dbl)
            n276 = local read "Measured_voltage(V)"() -> (w481:dbl)
            n277 = local read "Cur. Eff. (cd/A)"() -> (w478:dbl)
            n278 = local read "Lum.(cd/m2)"() -> (w480:dbl)
            n279 = local read "Lum/Lum0"() -> (w479:dbl)
            n280 = local read "Power(W)"() -> (w470:dbl)
            n281 = local read "Time (s)"() -> (w473:dbl)
            n282 = local read "EQE (%)"() -> (w476:dbl)
            n283 = local read "data path"() -> (w474:path)
            n284 = Build Array(w473, w472, w471, w481, w480, w479, w478, w477, w476, w470) -> (w475:dbl[])
            n285 = call-poly <vilib>:"Write To Spreadsheet File.vi"("delimiter (\\t)"="\t" ("delimiter (\\t)"), "transpose? (no:F)"=FALSE, "format (%.3f)"="%6e", "append to file? (new file:F)"=TRUE, "1D data"=w475, "file path (dialog if empty)"=w474) -> ()  [unwired: 1 in, 2 out]
          }
          frame #6 {
            n286 = local read "Current density (mA/cm2)"() -> (w502:dbl)
            n287 = local read "Lum. Pow. Eff. (lm/W)"() -> (w513:dbl)
            n288 = local read "Measured_Current(A)"() -> (w510:dbl)
            n289 = local read "Measured_voltage(V)"() -> (w509:dbl)
            n290 = local read "Cur. Eff. (cd/A)"() -> (w512:dbl)
            n291 = local read "Lum.(cd/m2)"() -> (w508:dbl)
            n292 = local read "Lum/Lum0"() -> (w507:dbl)
            n293 = local read "Power(W)"() -> (w503:dbl)
            n294 = local read "Time (s)"() -> (w511:dbl)
            n295 = local read "EQE (%)"() -> (w514:dbl)
            n296 = Number To Exponential String(number=w511) -> (E-format string=w515:string)  [unwired: 3 in]
            n297 = Number To Exponential String(number=w510) -> (E-format string=w516:string)  [unwired: 3 in]
            n298 = Number To Exponential String(number=w502) -> (E-format string=w506:string)  [unwired: 3 in]
            n299 = Number To Exponential String(number=w509) -> (E-format string=w517:string)  [unwired: 3 in]
            n300 = Number To Exponential String(number=w508) -> (E-format string=w518:string)  [unwired: 3 in]
            n301 = Number To Exponential String(number=w507) -> (E-format string=w519:string)  [unwired: 3 in]
            n302 = Number To Exponential String(number=w512) -> (E-format string=w520:string)  [unwired: 3 in]
            n303 = Number To Exponential String(number=w513) -> (E-format string=w521:string)  [unwired: 3 in]
            n304 = Number To Exponential String(number=w514) -> (E-format string=w522:string)  [unwired: 3 in]
            n305 = Number To Exponential String(number=w503) -> (E-format string=w505:string)  [unwired: 3 in]
            n306 = Build Array (concatenate)(w525, w520) -> (w489:string[])
            "CE array" <- w489
            n307 = Build Array (concatenate)(w530, w515) -> (w486:string[])
            "time array" <- w486
            n308 = Build Array (concatenate)(w529, w516) -> (w500:string[])
            "current array" <- w500
            n309 = Build Array (concatenate)(w501, w506) -> (w499:string[])
            "CurDen array" <- w499
            n310 = Build Array (concatenate)(w527, w518) -> (w488:string[])
            "Lum array" <- w488
            n311 = Build Array (concatenate)(w526, w519) -> (w487:string[])
            "L/L0 array" <- w487
            n312 = Build Array (concatenate)(w524, w521) -> (w490:string[])
            "LPE array" <- w490
            n313 = Build Array (concatenate)(w523, w522) -> (w491:string[])
            "EQE array" <- w491
            n314 = Build Array (concatenate)(w528, w517) -> (w498:string[])
            "voltage array" <- w498
            n315 = Build Array (concatenate)(w504, w505) -> (w492:string[])
            "power array" <- w492
            n316 = case shown="4" "Ring" {
              tunnel: [w531 w532 w533 w534 w535 w536] -> w497
              tunnel: w492 -> [_ _ _ _ _ w536]
              tunnel: w491 -> [_ _ _ _ w535 _]
              tunnel: w490 -> [_ _ _ w534 _ _]
              tunnel: w489 -> [_ _ w533 _ _ _]
              tunnel: w488 -> [_ w532 _ _ _ _]
              tunnel: w487 -> [w531 _ _ _ _ _]
              frame ..0 {
              }
              frame 1 {
              }
              frame 2 {
              }
              frame 3 {
              }
              frame 4 {
              }
              frame 5.. {
              }
            }
            n317 = Fract/Exp String To Number(string=w486) -> (number=w494:dbl[])  [unwired: 3 in, 1 out]
            n318 = Fract/Exp String To Number(string=w497) -> (number=w493:dbl[])  [unwired: 3 in, 1 out]
            n319 = Bundle(w494, w493) -> (→"Graph":cluster{dbl[], dbl[]})  [unwired: 1 in]
          }
        }
        n320 = local read "Interval (s)"() -> (w334:u32)
        n321 = Multiply(x=w334, y=u32 1000) -> (x*y=w339:u32)
        n322 = Wait (ms)(milliseconds to wait=w339) -> ()  [unwired: 1 out]
        n323 = local read "Auto stop"() -> (w317:bool)
        n324 = case shown="True" "stop" {
          frame False {
          }
          frame True {
            n325 = local write "Status"("Stopping measurement...Please wait..." ("Status")) -> ()
          }
        }
        n326 = case shown="True" w317 {
          tunnel: [FALSE w344] -> w335
          tunnel: w312 -> [_ w342]
          frame False {
          }
          frame True {
            n327 = local read "Ratio for auto stop"() -> (w343:dbl)
            n328 = Less Or Equal?(x=w342, y=w343) -> (x <= y?=w344:bool)
          }
        }
        n329 = Or(x=w335, y="stop") -> (x .or. y?=w336:bool)
      }
    }
    frame #5 {
      n330 = local read "VISA resource name out"() -> (w545:refnum<visa-resource-name>)
      n331 = local read "Wrapper Out"() -> (w546:u64)
      n332 = local read "Node Out"() -> (w542:string)
      n333 = local read "error out"() -> (w543:errorcluster)
      n334 = local write "Spectrometer"(FALSE ("Spectrometer")) -> ()
      n335 = call "Wrapper_closeAllSpectrometers.vi"("Wrapper In"=w546) -> ("Wrapper Out"=w547:u64)
      n336 = local write "Detector Saturated"(FALSE ("Det.Sat.")) -> ()
      n337 = local write "Keithley"(FALSE ("Keithley")) -> ()
      n338 = call "Wrapper_Destroy.vi"("Wrapper"=w547) -> ()
      n339 = call <instrlib>:"Source Output Enable.vi"("Output (Off)"=FALSE, "error in (no error)"=w543, "Channel (Channel A)"=Channel."Channel A", "Node In"=w542, "VISA resource name"=w545) -> ("error out"=w548:errorcluster, "Node Out"=w541:string, "VISA resource name out"=w549:refnum<visa-resource-name>)  [unwired: 4 out]
      n340 = local write "Status"("Measurement completed." ("Status")) -> ()
      n341 = call <instrlib>:"Close.vi"("error in (no error)"=w548, "VISA resource name"=w549) -> ()  [unwired: 10 out]
      n342 = local write "Node Out"(w541) -> ()
    }
  }
